vi "FileFGV.vi"(0 "File FGV 상태":enum16{"열기", "쓰기", "닫기"}(ring), 1 "배열":dbl[][](array[numeric]), 2 "파일 경로":path) -> ()   [LabVIEW 2020]
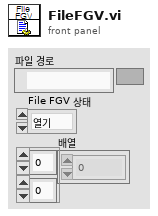
[diagram p1: front panel]
types:
  T1 = enum16{"open", "open or create", "create or replace", "create", "open (read-only)"}
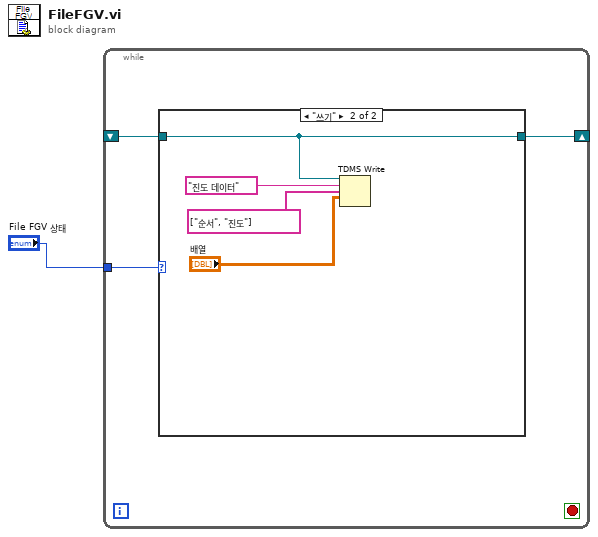
[diagram p0: block diagram]
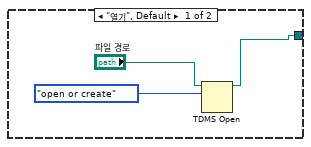
[diagram p2: hidden frame]
diagram:
  n1 = while {
    shift-right: [w3] -> _
    shift-left: _ -> [w2]
    tunnel: "File FGV 상태" -> [w4]
    stop <- _ stop-if-true
    n2 = case shown="\"쓰기\"" w4 {
      tunnel: [w5 w11] -> w3
      tunnel: w2 -> [_ w11]
      frame "열기", Default {
        n3 = TDMS Open(10:T1."open or create" ("동작(0:open)"), 11:"파일 경로") -> (3:w5:refnum<k34>)  [unwired: 5 in, 1 out]
      }
      frame "쓰기" {
        n4 = TDMS Write(0:w11, 5:"진도 데이터" ("그룹 이름 입력(제목없음)"), 7:string[] ["순서", "진도"] ("채널 이름 입력(제목없음)"), 9:"배열") -> ()  [unwired: 2 in, 4 out]
      }
    }
  }
